vi "FinalStateNode_New.vi"(0 "reference in":refnum<class "FinalStateNode.lvclass">, 1 "Object name":string, 5 "error in (no error)":errorcluster, 6 "GoopReferenceIn":T1, 8 "Create method":T2(ring)) -> (12 "GoopReferenceOut":T1, 14 "reference out":refnum<class "FinalStateNode.lvclass">, 16 "# of objects":i32, 19 "error out":errorcluster)   [LabVIEW 2014, in "FinalStateNode.lvclass"]
doc: "Looks up an existing FinalStateNode object matching object name or creates a new FinalStateNode object and returns a refnum you can use when calling other FinalStateNode methods.\n\nObjects created with this VI should be destroyed using the FinalStateNode Delete VI.\n\n[GOOP 2.0.15]"
uses:
  <resource>/Framework/Providers/Open_GDS/UML/FinalStateNode_class/FinalStateNode.lvclass
  <resource>/Framework/Providers/Open_GDS/UML/AbstractNode_class/ObjectReference.ctl
  <vilib>/addons/_goop3.llb/3GOOPStates.ctl
  <resource>/Framework/Providers/Open_GDS/UML/FinalStateNode_class/FinalStateNode.lvclass/FinalStateNode.ctl
  <resource>/Framework/Providers/Open_GDS/UML/AbstractNode_class/AbstractNode.lvclass
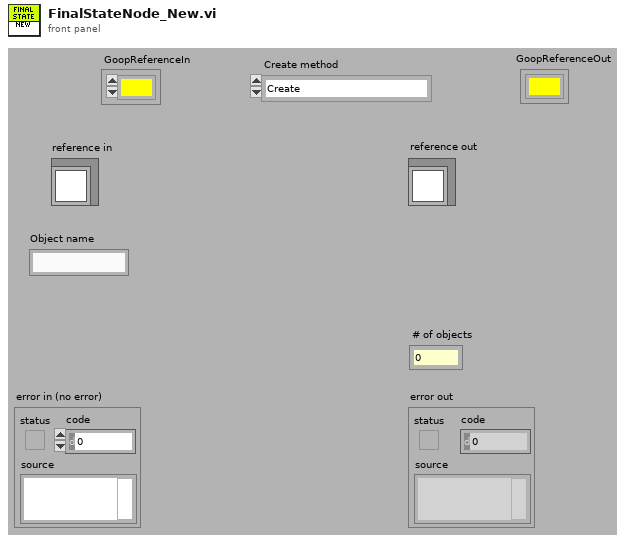
[diagram p1: front panel]
types:
  T1 = typedef "AbstractNode.lvclass/ObjectReference.ctl" = refnum<k1>
  T2 = enum16{"Create", "Create or look up existing", "Look up existing"}
  T3 = typedef "3GOOPStates.ctl" = enum16{"Set", "Get", "New", "Delete", "Clear", "Test and get", "Unlock data", "Information", "Look up existing", "New or look up existing", "Test and get shared", "Get shared", "Set shared", "Unlock shared", "Find dynamic method", "Register dynamic method", "Preload dynamic method", "Probe", "Cast to more generic", "Cast to more specific"}
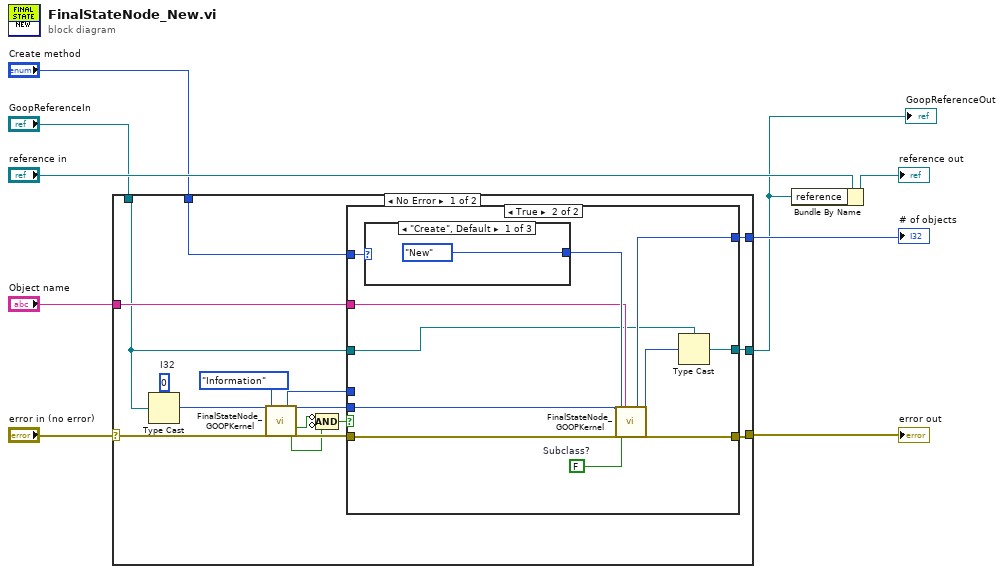
[diagram p0: block diagram]
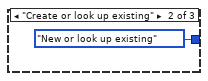
[diagram p3: hidden frame]
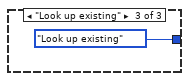
[diagram p4: hidden frame]
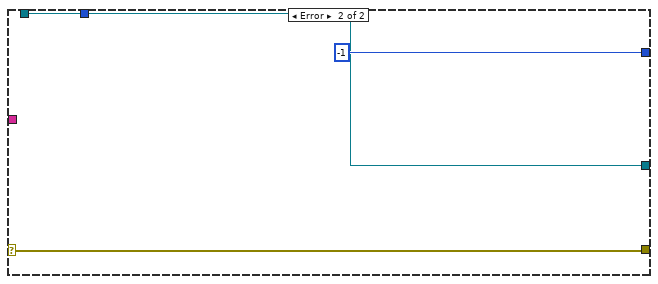
[diagram p5: hidden frame]
diagram:
  n1 = case shown="No Error" "error in (no error)" {
    selector: "error in (no error)" -> [w18 w44]
    tunnel: [w24 w43] -> w1
    tunnel: [w23 w44] -> w9
    tunnel: [w22 -1 ("Nr of open handles")] -> w8
    tunnel: "Object name" -> [w21 _]
    tunnel: "Create method" -> [w25 _]
    tunnel: "GoopReferenceIn" -> [w13 w43]
    frame No Error {
      w20 = 0  # I32
      n2 = Type Cast(type=w20, x=w13) -> (*(type *) &x=w14:i32)
      n3 = call <resource>:"FinalStateNode_GOOPKernel.vi"("Ref in"=w14, "error in (no error)"=w18, "Action"=3GOOPStates."Information") -> ("# of objects"=w12:i32, "IsSubclass?"=w17:bool, "Ref out"=w10:i32, "Exists?"=w16:bool, "error out"=w19:errorcluster)  [unwired: 12 in, 8 out]
      n4 = Compound Arithmetic op=AND(invert w16, invert w17) -> (w15:bool)
      n5 = case shown="True" w15 {
        tunnel: w25 -> [_ w39]
        tunnel: [w27 w38] -> w24
        tunnel: w19 -> [w28 w31]
        tunnel: [w28 w37] -> w23
        tunnel: [w26 w32] -> w22
        tunnel: w21 -> [_ w33]
        tunnel: w13 -> [w27 w29]
        tunnel: w12 -> [w26 _]
        tunnel: w10 -> [_ w30]
        frame False {
          # "Reference already exists and belongs to subclass."
        }
        frame True {
          w34 = FALSE  # Subclass?
          n6 = case shown="\"Create\", Default" w39 {
            tunnel: [3GOOPStates."New" ("Action") 3GOOPStates."New or look up existing" ("Action") 3GOOPStates."Look up existing" ("Action")] -> w36
            frame "Create", Default {
            }
            frame "Create or look up existing" {
            }
            frame "Look up existing" {
            }
          }
          n7 = call <resource>:"FinalStateNode_GOOPKernel.vi"("Ref in"=w30, "error in (no error)"=w31, "Action"=w36, "Subclass?"=w34, "Object name"=w33) -> ("# of objects"=w32:i32, "Ref out"=w35:i32, "error out"=w37:errorcluster)  [unwired: 10 in, 10 out]
          n8 = Type Cast(type=w29, x=w35) -> (*(type *) &x=w38:T1)
        }
      }
    }
    frame Error {
    }
  }
  "error out" <- w9
  "# of objects" <- w8
  "GoopReferenceOut" <- w1
  n9 = Bundle By Name(cluster="reference in", "reference"=w1) -> (→"reference out":refnum<class "FinalStateNode.lvclass">)
